vi "Read Write App Config.vi"(7 "Write (F)":bool, 8 "Error IN":errorcluster, 10 "App Config":T1={"Location"="", "Profiles Path"=path "", "Current Profile"="", "CA Number"="", "Cycles Completed"=0, "Controller Type:"=enum."Kuhnke", "Stagger Time (ms)"=0, "Tank 1 Fuel"="", "Tank 2 Fuel"="", "Serial Numbers"={"Position 1 SN"="", "Position 2 SN"="", "Poaition 3 SN"="", "Position 4 SN"="", "Position 5 SN"="", "Position 6 SN"=""}, "Pumps Present"={"Pump 1"=FALSE, "Pump 2"=FALSE, "Pump 3"=FALSE, "Pump 4"=FALSE, "Pump 5"=FALSE, "Pump 6"=FALSE}, "VoltCtrlRef"="", "VoltageSelect"=FALSE, "Watlow Present"=FALSE, "Temp 1"=0.0, "Temp 2"=0.0, "V_Run PI?"=FALSE, "Voltage Limits"={"V_Step"=1e-05, "V_CmdMax"=0.0, "V_CmdMin"=0.0}, "Voltage Far PI"={"V_FarSlew"=10.0, "V_FarKp"=0.0, "V_FarKi"=0.0}, "Voltage Mid PI"={"V_MidSlew"=10.0, "V_MidKp"=0.0, "V_MidKi"=0.0}, "Voltage Close PI"={"V_CloseSlew"=10.0, "V_CloseKp"=0.0, "V_CloseKi"=0.0}, "Voltage Scale"={"V_FFm"=0.0, "V_FFb"=0.0}, "Voltage Cutoffs"={"V_MidCutoff"=0.0, "V_CloseCutoff"=0.0}, "Pressure Scale"={"Pres_FFm"=1e-05, "Pres_FFb"=0.0}, "Temp Format"=0, "Temp Tolerance"=0.0, "Target Voltage"=0.0, "Target Pressure"=0.0, "Data Log Init"={"Data Path"=path "", "Data Log Rate (S/s)"=0, "AKLH Rate (Hours/S)"=0.0, "Sync Time Offset (min)"=0, "IP Last 3"=0, "WebDAV IP"=""}, "Email Handler IP"="", "ADC Check"=FALSE, "3 Pump Tank"=FALSE, "Cycle Threshold:"=3.0, "Cycle Pts to Avg:"=3, "Anomaly Threshold:"=3.0, "Normal Steps:"=3, "Step Threshold:"=3.0, "Network Drive IP"="", "Network Drive Password"="", "Bank 1 Offset"=0.0, "Bank 2 Offset"=0.0} {"Bank 2 Offset" min=0.0 max=999999.0 step=1.0; "Bank 1 Offset" min=0.0 max=999999.0 step=1.0; "Step Threshold:" min=0.0 max=999999.0 step=1.0; "Normal Steps:" max=999999 step=1; "Anomaly Threshold:" min=0.0 max=999999.0 step=1.0; "Cycle Pts to Avg:" max=999999 step=1; "Cycle Threshold:" min=0.0 max=999999.0 step=1.0}, 11 "Refnum in":T4) -> (0 "Error OUT":errorcluster, 2 "App Config OUT":T1={"Location"="", "Profiles Path"=path "", "Current Profile"="", "CA Number"="", "Cycles Completed"=0, "Controller Type:"=enum."Kuhnke", "Stagger Time (ms)"=0, "Tank 1 Fuel"="", "Tank 2 Fuel"="", "Serial Numbers"={"Position 1 SN"="", "Position 2 SN"="", "Poaition 3 SN"="", "Position 4 SN"="", "Position 5 SN"="", "Position 6 SN"=""}, "Pumps Present"={"Pump 1"=FALSE, "Pump 2"=FALSE, "Pump 3"=FALSE, "Pump 4"=FALSE, "Pump 5"=FALSE, "Pump 6"=FALSE}, "VoltCtrlRef"="", "VoltageSelect"=FALSE, "Watlow Present"=FALSE, "Temp 1"=0.0, "Temp 2"=0.0, "V_Run PI?"=FALSE, "Voltage Limits"={"V_Step"=1e-05, "V_CmdMax"=0.0, "V_CmdMin"=0.0}, "Voltage Far PI"={"V_FarSlew"=10.0, "V_FarKp"=0.0, "V_FarKi"=0.0}, "Voltage Mid PI"={"V_MidSlew"=10.0, "V_MidKp"=0.0, "V_MidKi"=0.0}, "Voltage Close PI"={"V_CloseSlew"=10.0, "V_CloseKp"=0.0, "V_CloseKi"=0.0}, "Voltage Scale"={"V_FFm"=0.0, "V_FFb"=0.0}, "Voltage Cutoffs"={"V_MidCutoff"=0.0, "V_CloseCutoff"=0.0}, "Pressure Scale"={"Pres_FFm"=1e-05, "Pres_FFb"=0.0}, "Temp Format"=0, "Temp Tolerance"=0.0, "Target Voltage"=0.0, "Target Pressure"=0.0, "Data Log Init"={"Data Path"=path "", "Data Log Rate (S/s)"=0, "AKLH Rate (Hours/S)"=0.0, "Sync Time Offset (min)"=0, "IP Last 3"=0, "WebDAV IP"=""}, "Email Handler IP"="", "ADC Check"=FALSE, "3 Pump Tank"=FALSE, "Cycle Threshold:"=3.0, "Cycle Pts to Avg:"=3, "Anomaly Threshold:"=3.0, "Normal Steps:"=3, "Step Threshold:"=3.0, "Network Drive IP"="", "Network Drive Password"="", "Bank 1 Offset"=0.0, "Bank 2 Offset"=0.0} {"Bank 2 Offset" min=0.0 max=999999.0 step=1.0; "Bank 1 Offset" min=0.0 max=999999.0 step=1.0; "Step Threshold:" min=0.0 max=999999.0 step=1.0; "Normal Steps:" max=999999 step=1; "Anomaly Threshold:" min=0.0 max=999999.0 step=1.0; "Cycle Pts to Avg:" max=999999 step=1; "Cycle Threshold:" min=0.0 max=999999.0 step=1.0}, 3 "Refnum out":T4)   [LabVIEW 2019]
uses:
  <vilib>/Utility/config.llb/Config Data RefNum.ctl
  Type Defs/App Config.ctl
  Type Defs/Controller Names.ctl
  Data Logger/Data Log Init.ctl
  <vilib>/Utility/config.llb/NI_LVConfig.lvlib
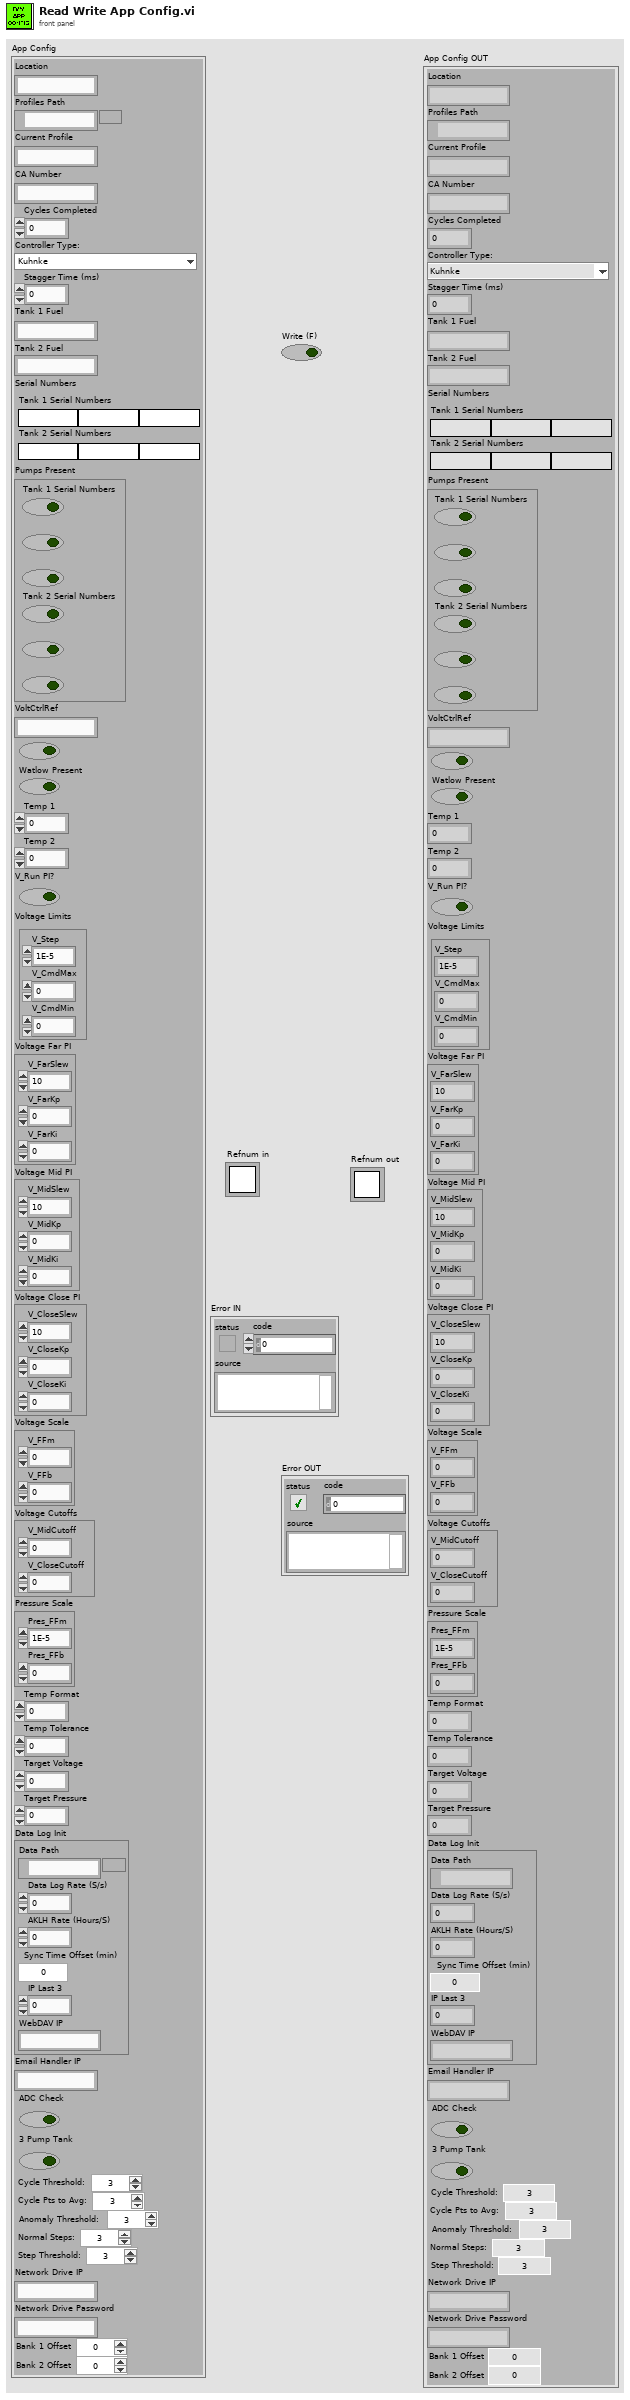
[diagram p1: front panel]
types:
  T1 = typedef "App Config.ctl" = cluster{"Location":string, "Profiles Path":path, "Current Profile":string, "CA Number":string, "Cycles Completed":u32, "Controller Type:":T2, "Stagger Time (ms)":i32, "Tank 1 Fuel":string, "Tank 2 Fuel":string, "Serial Numbers":cluster{"Position 1 SN":string, "Position 2 SN":string, "Poaition 3 SN":string, "Position 4 SN":string, "Position 5 SN":string, "Position 6 SN":string}, "Pumps Present":cluster{"Pump 1":bool, "Pump 2":bool, "Pump 3":bool, "Pump 4":bool, "Pump 5":bool, "Pump 6":bool}, "VoltCtrlRef":string, "VoltageSelect":bool, "Watlow Present":bool, "Temp 1":dbl, "Temp 2":dbl, "V_Run PI?":bool, "Voltage Limits":cluster{"V_Step":dbl, "V_CmdMax":dbl, "V_CmdMin":dbl}, "Voltage Far PI":cluster{"V_FarSlew":dbl, "V_FarKp":dbl, "V_FarKi":dbl}, "Voltage Mid PI":cluster{"V_MidSlew":dbl, "V_MidKp":dbl, "V_MidKi":dbl}, "Voltage Close PI":cluster{"V_CloseSlew":dbl, "V_CloseKp":dbl, "V_CloseKi":dbl}, "Voltage Scale":cluster{"V_FFm":dbl, "V_FFb":dbl}, "Voltage Cutoffs":cluster{"V_MidCutoff":dbl, "V_CloseCutoff":dbl}, "Pressure Scale":cluster{"Pres_FFm":dbl, "Pres_FFb":dbl}, "Temp Format":i32, "Temp Tolerance":dbl, "Target Voltage":dbl, "Target Pressure":dbl, "Data Log Init":T3, "Email Handler IP":string, "ADC Check":bool, "3 Pump Tank":bool, "Cycle Threshold:":dbl, "Cycle Pts to Avg:":i32, "Anomaly Threshold:":dbl, "Normal Steps:":u32, "Step Threshold:":dbl, "Network Drive IP":string, "Network Drive Password":string, "Bank 1 Offset":dbl, "Bank 2 Offset":dbl}
  T2 = typedef "Controller Names.ctl" = enum16{"Kuhnke", "Helbako BLDC", "Conti", "Hella BLDC OL PWM", "Hella BLDC Turbine OL PWM", "Hella BLDC Pressure", "Helbako (old)", "TI PWM", "PSA", "Hella Gas", "Hella Diesel", "8 Comm", "10 Comm", "8 Comm Hella", "10 Comm Hella", "8 Comm Omron", "10 Comm Omron", "8 Comm Nissan", "10 Comm Nissan"}
  T3 = typedef "Data Log Init.ctl" = cluster{"Data Path":path, "Data Log Rate (S/s)":u32, "AKLH Rate (Hours/S)":dbl, "Sync Time Offset (min)":i32, "IP Last 3":i32, "WebDAV IP":string}
  T4 = typedef "NI_LVConfig.lvlib/Config Data RefNum.ctl" = refnum<k1>
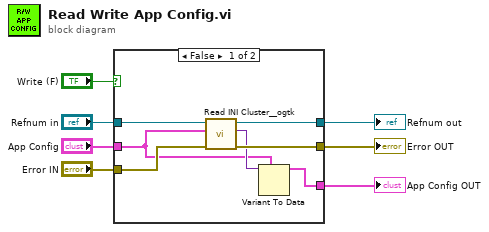
[diagram p0: block diagram]
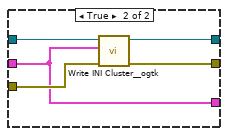
[diagram p2: hidden frame]
diagram:
  n1 = case shown="False" "Write (F)" {
    tunnel: "Refnum in" -> [w14 w19]
    tunnel: "App Config" -> [w10 w16]
    tunnel: "Error IN" -> [w13 w18]
    tunnel: [w8 w17] -> w2
    tunnel: [w9 w16] -> w4
    tunnel: [w12 w15] -> w3
    frame False {
      n2 = call <userlib>:"Read INI Cluster__ogtk.vi"("error in (no error)"=w13, "INI Fomatted Cluster Type"=w10, "refnum"=w14) -> ("error out"=w12:errorcluster, "INI Fomatted Cluster"=w11:variant, "dup refnum"=w8:T4)  [unwired: 4 in, 2 out]
      n3 = Variant To Data(type=w10, Variant=w11) -> (data=w9:T1)  [unwired: 1 in, 1 out]
    }
    frame True {
      n4 = call <userlib>:"Write INI Cluster__ogtk.vi"("error in (no error)"=w18, "INI Fomatted Cluster"=w16, "refnum"=w19) -> ("error out"=w15:errorcluster, "dup refnum"=w17:T4)  [unwired: 7 in]
    }
  }
  "Error OUT" <- w3
  "Refnum out" <- w2
  "App Config OUT" <- w4
